vi "TilePlot_auto.vi"(0 "Array":dbl[][](array[numeric]), 2 "Label":string, 3 "Colormap":T2, 4 "Line Color":T1=2147483647 items=["Automatic"=2147483647, "Black"=0, "White"=16777215, "Red"=16711680, "Green"=2263842, "Blue"=255, "Cyan"=65535, "Magenta"=16711935, "Yellow"=16776960], 5 "Line Width":sgl=nan) -> (14 "Tile Plot":picture)   [LabVIEW 2014]
uses:
  <vilib>/Heliosphere Research LLC/Advanced Plotting Toolkit/properties/Colormap_Map.ctl
  <vilib>/Heliosphere Research LLC/Advanced Plotting Toolkit/typedefs/PlotColor.ctl
  <vilib>/Heliosphere Research LLC/Advanced Plotting Toolkit/api_plotting/TilesProperties.ctl
  <vilib>/Heliosphere Research LLC/Advanced Plotting Toolkit/properties/Colormap.ctl
  <vilib>/Heliosphere Research LLC/Advanced Plotting Toolkit/properties/Colormap_Scaling.ctl
  <vilib>/Heliosphere Research LLC/Advanced Plotting Toolkit/properties/Line.ctl
  <vilib>/Heliosphere Research LLC/Advanced Plotting Toolkit/properties/Line_Style.ctl
  <vilib>/Heliosphere Research LLC/Advanced Plotting Toolkit/properties/Display.ctl
  <vilib>/Heliosphere Research LLC/Advanced Plotting Toolkit/Advanced Plotting Toolkit.lvlib
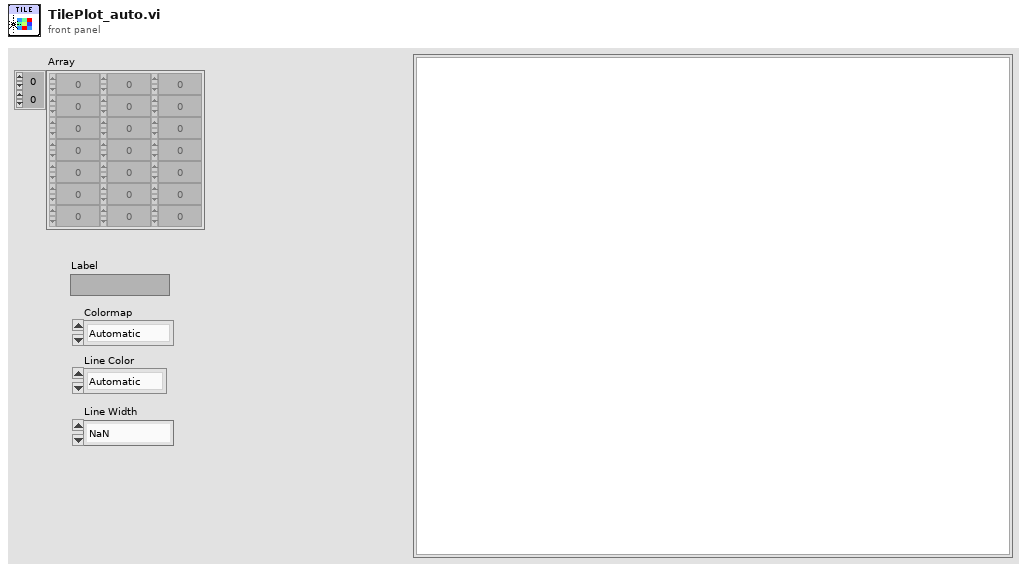
[diagram p1: front panel]
types:
  T1 = typedef "Advanced Plotting Toolkit.lvlib/PlotColor.ctl" = u32
  T2 = typedef "Advanced Plotting Toolkit.lvlib/Colormap_Map.ctl" = enum16{"Automatic", "Rainbow", "Hot and Cold", "White-Black", "White-Blue", "White-Green", "White-Red", "Fire", "Water", "Earth", "Air", "Pastel", "Banded", "Stepped"}
  T3 = typedef "Advanced Plotting Toolkit.lvlib/TilesProperties.ctl" = cluster{"Colormap":T4, "Line":T6, "Display":T8}
  T4 = typedef "Advanced Plotting Toolkit.lvlib/Colormap.ctl" = cluster{"Map":T2, "Value Min":dbl, "Value Max":dbl, "Scaling":T5, "Reverse":bool}
  T5 = typedef "Advanced Plotting Toolkit.lvlib/Colormap_Scaling.ctl" = enum16{"Default"}
  T6 = typedef "Advanced Plotting Toolkit.lvlib/Line.ctl" = cluster{"Style":T7, "Color":T1, "Width":sgl}
  T7 = typedef "Advanced Plotting Toolkit.lvlib/Line_Style.ctl" = enum16{"Automatic", "Solid", "Dashed", "Dotted", "Dash-dot", "Invisible"}
  T8 = typedef "Advanced Plotting Toolkit.lvlib/Display.ctl" = cluster{"Alpha":dbl, "Z Order":dbl}
  T9 = typedef "Advanced Plotting Toolkit.lvlib/PlotID.ctl" = i32
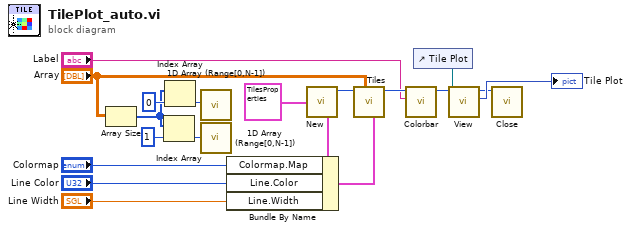
[diagram p0: block diagram]
diagram:
  n1 = Array Size(array="Array") -> (size(s)=w4:i32[])
  n2 = Index Array(array=w4, index=1) -> (element=w2:i32)
  n3 = Index Array(array=w4, index=0) -> (element=w3:i32)
  n4 = call "1D Array (Range[0,N-1]).vi"("Range"=w3) -> ()  [unwired: 18 in, 1 out]
  n5 = call "1D Array (Range[0,N-1]).vi"("Range"=w2) -> ()  [unwired: 18 in, 1 out]
  n6 = Bundle By Name(cluster=T3 {"Colormap"={"Map"=enum."Automatic", "Value Min"=nan, "Value Max"=nan, "Scaling"=enum."Default", "Reverse"=FALSE}, "Line"={"Style"=enum."Automatic", "Color"=2147483647, "Width"=nan}, "Display"={"Alpha"=nan, "Z Order"=nan}} ("Properties"), "Colormap.Map"="Colormap", "Line.Color"="Line Color", "Line.Width"="Line Width") -> (w13:T3)
  n7 = call <vilib>:"New.vi"() -> ("Plot ID"=w15:T9)  [unwired: 10 in, 1 out]
  n8 = call <vilib>:"Tiles.vi"("Properties"=w13, "Z Data"="Array", "Plot ID"=w15) -> ("Plot ID Out"=w11:T9)  [unwired: 7 in, 1 out]
  n9 = call <vilib>:"Colorbar.vi"("Label"="Label", "Plot ID"=w11) -> ("Plot ID Out"=w10:T9)  [unwired: 8 in, 1 out]
  n10 = control-ref of="Tile Plot"() -> (w17:refnum<vi>)
  n11 = call <vilib>:"View.vi"("Ref for Sizing"=w17, "Plot ID"=w10) -> ("Picture"=→"Tile Plot":picture, "Plot ID Out"=w16:T9)  [unwired: 7 in, 1 out]
  n12 = call <vilib>:"Close.vi"("Plot ID"=w16) -> ()  [unwired: 10 in, 1 out]
